vi "Generate default line from name.vi"(10 "Name":string, 11 "Multiplexer configuration in":refnum<class "Multiplexer configuration.lvclass">) -> (3 "Line":T1)   [LabVIEW 2021, in "Multiplexer editor node.lvclass"]
uses:
  Multiplexer editor node.lvclass
  configuration/Multiplexer configuration.lvclass
  configuration/Line.ctl
  <vilib>/NI/Tag Bus Module Framework/channel/TBM channel.lvclass
  C:/Program Files (x86)/National Instruments/LabVIEW 2021/vi.lib/NI/Tag Bus/tag/tag descriptor.lvclass
  <vilib>/NI/Tag Bus/tag/Data Type.ctl
  configuration/permissions.ctl
  <vilib>/NI/Tag Bus/tag/tag descriptor.lvclass/tag descriptor.ctl
  <vilib>/NI/Tag Bus/tag/read tag name.vi
  <vilib>/NI/Tag Bus/tag/tag descriptor.lvclass
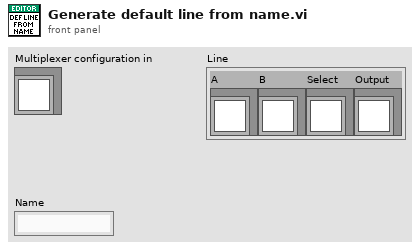
[diagram p1: front panel]
types:
  T1 = typedef "Multiplexer configuration.lvclass/Line.ctl" = cluster{"A":refnum<class "TBM channel.lvclass">, "B":refnum<class "TBM channel.lvclass">, "Select":refnum<class "TBM channel.lvclass">, "Output":refnum<class "TBM channel.lvclass">}
  T2 = typedef "Multiplexer configuration.lvclass/permissions.ctl" = enum32{"Read from HW", "Write to HW"}
  T3 = typedef "tag bus.lvlib/tag descriptor.lvclass/Data Type.ctl" = enum16{"Double", "Single", "I64", "I32", "I16", "I8", "U64", "U32", "U16", "U8", "Boolean", "String", "Array of Double", "Array of Single", "Array of I64", "Array of I32", "Array of I16", "Array of I8", "Array of U64", "Array of U32", "Array of U16", "Array of U8", "Array of Boolean", "Array of String"}
  T4 = typedef "TBM channel.lvclass/channel classification.ctl" = enum16{"input data", "output data", "processing parameter", "processing result"}
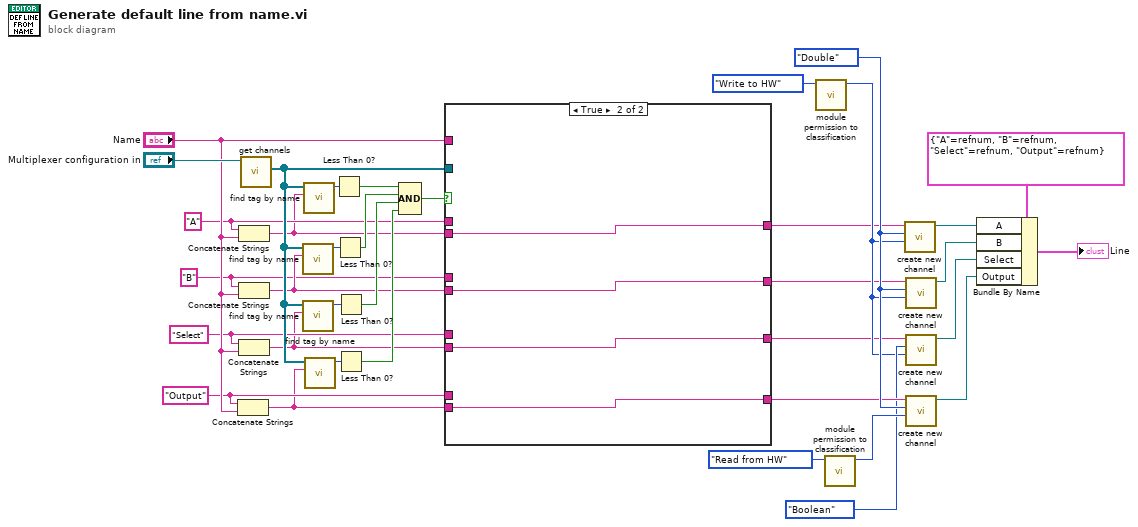
[diagram p0: block diagram]
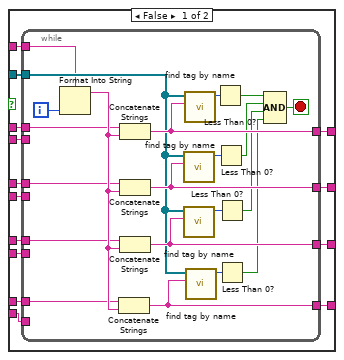
[diagram p2: hidden frame]
diagram:
  w3 = "Output" ("string")
  w5 = "Select" ("string")
  w6 = "B" ("string")
  w9 = "A" ("string")
  w34 = Data_Type."Double" ("data type")
  n1 = Concatenate Strings(w3, "Name") -> (w2:string)
  n2 = Concatenate Strings(w9, "Name") -> (w8:string)
  n3 = Concatenate Strings(w6, "Name") -> (w7:string)
  n4 = Concatenate Strings(w5, "Name") -> (w4:string)
  n5 = call-dynamic "get channels.vi"("Multiplexer configuration in"="Multiplexer configuration in") -> ("channels"=w14:refnum<class "TBM channel.lvclass">[])  [unwired: 9 in, 1 out]
  n6 = call <vilib>:"find tag by name.vi"("name"=w7, "tags in"=w14) -> ("index"=w18:i32)  [unwired: 9 in]
  n7 = call <vilib>:"find tag by name.vi"("name"=w4, "tags in"=w14) -> ("index"=w17:i32)  [unwired: 9 in]
  n8 = call <vilib>:"find tag by name.vi"("name"=w8, "tags in"=w14) -> ("index"=w19:i32)  [unwired: 9 in]
  n9 = call <vilib>:"find tag by name.vi"("name"=w2, "tags in"=w14) -> ("index"=w16:i32)  [unwired: 9 in]
  n10 = Less Than 0?(x=w19) -> (x < 0?=w13:bool)
  n11 = Less Than 0?(x=w18) -> (x < 0?=w12:bool)
  n12 = Less Than 0?(x=w17) -> (x < 0?=w11:bool)
  n13 = Less Than 0?(x=w16) -> (x < 0?=w10:bool)
  n14 = Compound Arithmetic op=AND(w13, w12, w11, w10) -> (w1:bool)
  n15 = case shown="True" w1 {
    tunnel: [w50 w72] -> w32
    tunnel: [w49 w73] -> w28
    tunnel: [w48 w74] -> w27
    tunnel: [w47 w75] -> w25
    tunnel: "Name" -> [w46 _]
    tunnel: w14 -> [w45 _]
    tunnel: w9 -> [w44 _]
    tunnel: w8 -> [w43 w75]
    tunnel: w7 -> [w42 w74]
    tunnel: w6 -> [w41 _]
    tunnel: w5 -> [w40 _]
    tunnel: w4 -> [w39 w73]
    tunnel: w3 -> [w38 _]
    tunnel: w2 -> [w37 w72]
    frame False {
      n16 = while {
        tunnel: [w69] -> w47
        tunnel: w45 -> [w64]
        tunnel: [w68] -> w48
        tunnel: [w66] -> w49
        tunnel: [w56] -> w50
        tunnel: w46 -> [w55]
        tunnel: w44 -> [w54]
        tunnel: w43 -> [_]
        tunnel: w42 -> [_]
        tunnel: w41 -> [w53]
        tunnel: w40 -> [w52]
        tunnel: w39 -> [_]
        tunnel: w38 -> [w51]
        tunnel: w37 -> [_]
        i -> [w71]
        stop <- w58 stop-if-true
        n17 = Format Into String(format string=w55, w71) -> (resulting string=w57:string)  [unwired: 2 in, 1 out]
        n18 = Concatenate Strings(w51, w57) -> (w56:string)
        n19 = Concatenate Strings(w54, w57) -> (w69:string)
        n20 = Concatenate Strings(w53, w57) -> (w68:string)
        n21 = Concatenate Strings(w52, w57) -> (w66:string)
        n22 = call <vilib>:"find tag by name.vi"("name"=w68, "tags in"=w64) -> ("index"=w67:i32)  [unwired: 9 in]
        n23 = call <vilib>:"find tag by name.vi"("name"=w66, "tags in"=w64) -> ("index"=w65:i32)  [unwired: 9 in]
        n24 = call <vilib>:"find tag by name.vi"("name"=w69, "tags in"=w64) -> ("index"=w70:i32)  [unwired: 9 in]
        n25 = call <vilib>:"find tag by name.vi"("name"=w56, "tags in"=w64) -> ("index"=w63:i32)  [unwired: 9 in]
        n26 = Less Than 0?(x=w70) -> (x < 0?=w62:bool)
        n27 = Less Than 0?(x=w67) -> (x < 0?=w61:bool)
        n28 = Less Than 0?(x=w65) -> (x < 0?=w60:bool)
        n29 = Less Than 0?(x=w63) -> (x < 0?=w59:bool)
        n30 = Compound Arithmetic op=AND(w62, w61, w60, w59) -> (w58:bool)
      }
    }
    frame True {
    }
  }
  n31 = call "module permission to classification.vi"("display permissions"=permissions."Write to HW") -> ("channel classification"=w29:T4)  [unwired: 10 in]
  n32 = call "module permission to classification.vi"("display permissions"=permissions."Read from HW") -> ("channel classification"=w36:T4)  [unwired: 10 in]
  n33 = call <vilib>:"create new channel.vi"("channel classification"=w29, "data type"=w34, "channel name"=w25) -> ("channel"=w21:refnum<class "TBM channel.lvclass">)  [unwired: 8 in]
  n34 = call <vilib>:"create new channel.vi"("channel classification"=w29, "data type"=w34, "channel name"=w27) -> ("channel"=w26:refnum<class "TBM channel.lvclass">)  [unwired: 8 in]
  n35 = call <vilib>:"create new channel.vi"("channel classification"=w29, "data type"=Data_Type."Boolean", "channel name"=w28) -> ("channel"=w31:refnum<class "TBM channel.lvclass">)  [unwired: 8 in]
  n36 = call <vilib>:"create new channel.vi"("channel classification"=w36, "data type"=w34, "channel name"=w32) -> ("channel"=w33:refnum<class "TBM channel.lvclass">)  [unwired: 8 in]
  n37 = Bundle By Name(cluster=T1 {"A"=refnum, "B"=refnum, "Select"=refnum, "Output"=refnum} ("Line"), "A"=w21, "B"=w26, "Select"=w31, "Output"=w33) -> (→"Line":T1)
